vi "AddDependency.vi"(8 "error in (no error)":errorcluster, 9 "Level":string, 10 "Dependency":refnum<class "SMO.lvclass">, 11 "SMO in":refnum<class "SMO.lvclass">) -> (0 "error out":errorcluster, 3 "SMO out":refnum<class "SMO.lvclass">)   [LabVIEW 2013, in "SMO.lvclass"]
uses:
  SMO.lvclass
  Typedefs/SMO Dependency--Cluster.ctl
  Typedefs/SMO Dependency Event--Cluster.ctl
  Typedefs/SMO Dependency Event--Enum.ctl
  SMO.lvclass/SMO.ctl
  <vilib>/regexp/Match Regular Expression.xnode
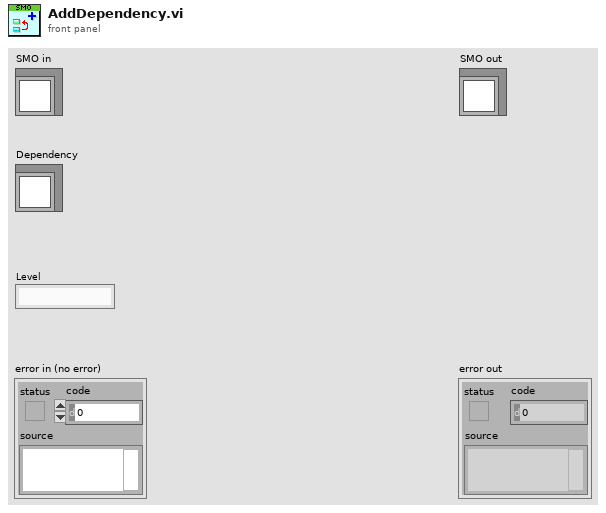
[diagram p1: front panel]
types:
  T1 = typedef "SMO.lvclass/SMO Dependency Event--Cluster.ctl" = cluster{"Name":string, "GUID":string, "Event":T2}
  T2 = typedef "SMO.lvclass/SMO Dependency Event--Enum.ctl" = enum16{"Added", "Removed", "Started", "Stopped"}
  T3 = typedef "SMO.lvclass/SMO Dependency--Cluster.ctl" = cluster{"Dependency":refnum<class "SMO.lvclass">, "Level":string}
  T4 = typedef "SMO.lvclass/PrivateData--Ref.ctl" = refnum<data-value>
  T5 = typedef "SMO.lvclass/PrivateData--Cluster.ctl" = cluster{"Parent Call":T6, "Registered Processes":T7[], "Sync Notifier":refnum<notifier>, "Process Error Notifier":refnum<notifier>, "Protected Events":T8, "Public Events":T9, "SMO State":T10, "[Dependencies]":T3[], "[Attributes]":refnum<class "Attribute.lvclass">[], "Launcher Close":refnum<notifier>, "Caller Watchdog":refnum<queue>}
  T6 = typedef "SMO.lvclass/Parent Call--Enum.ctl" = enum16{"Allows parent to run", "Does not request parent to run"}
  T7 = typedef "SMO.lvclass/RegisteredProcessData--Cluster.ctl" = cluster{"Name":string, "Static VI Ref":refnum<vi>, "Running":bool, "NotifierRef":u32}
  T8 = typedef "SMO.lvclass/Protected Events.ctl" = cluster{"StopProcesses":refnum<user-event>, "AbortProcesses":refnum<user-event>, "Config Changed":refnum<user-event>, "Dependency":refnum<user-event>}
  T9 = typedef "SMO.lvclass/Public Events.ctl" = cluster{"Error":refnum<user-event>, "State":refnum<user-event>}
  T10 = typedef "SMO.lvclass/SMOState --Enum.ctl" = enum16{"unknown", "Created", "Started", "Stopped"}
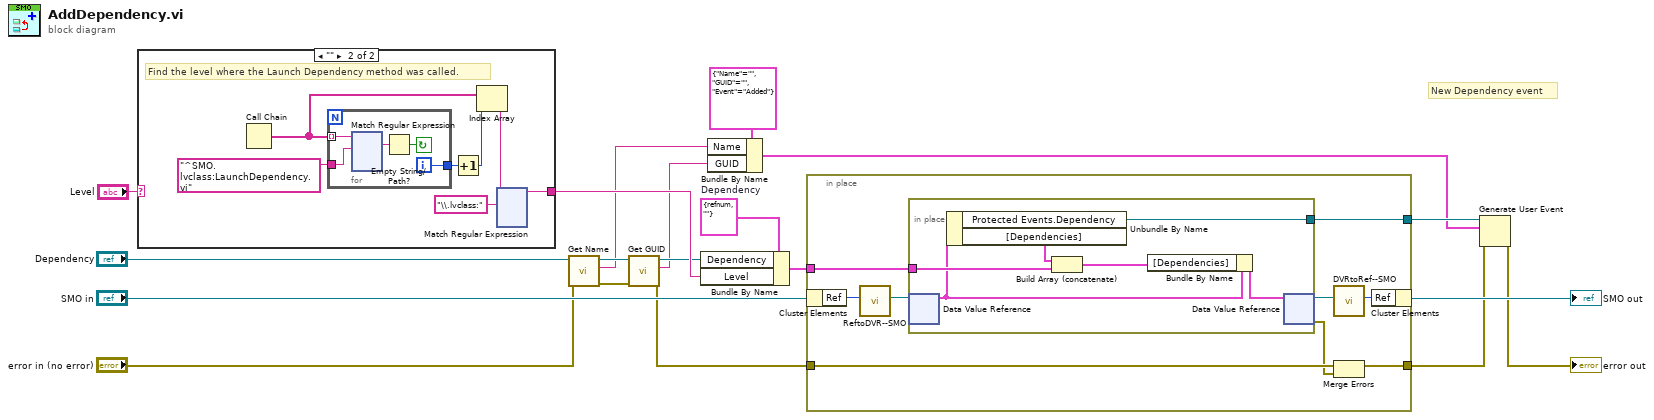
[diagram p0: block diagram]
diagram:
  w18 = T3 {"Dependency"=refnum, "Level"=""}  # Dependency
  # "New Dependency event"
  n1 = case shown="\"\"" "Level" {
    selector: "Level" -> [w20 _]
    tunnel: [w20 w21] -> w16
    frame Default {
    }
    frame "" {
      # "Find the level where the Launch Dependency method was called."
      n2 = Call Chain() -> (call chain=w26:string[])
      n3 = for {
        tunnel: w26 -> [w146] mode=indexing
        tunnel: "^SMO.lvclass:LaunchDependency.vi" -> [w145]
        tunnel: [w142] -> w25
        i -> [w142]
        stop <- w143 continue-if-true
        n4 = xnode "Match Regular Expression"("input string"=w146, "regular expression"=w145) -> ("whole match"=w144:string)  [unwired: 4 in, 4 out]
        n5 = Empty String/Path?(string/path=w144) -> (empty?=w143:bool)
      }
      n6 = Increment(x=w25) -> (x+1=w24:i32)
      n7 = Index Array(array=w26, index=w24) -> (element=w23:string)
      n8 = xnode "Match Regular Expression"("input string"=w23, "regular expression"="\\.lvclass:") -> ("before match"=w21:string)  [unwired: 4 in, 4 out]
    }
  }
  n9 = call "Get Name.vi"("error in (no error)"="error in (no error)", "SMO"="Dependency") -> ("error out"=w8:errorcluster, "Name"=w3:string, "SMO out"=w10:refnum<class "SMO.lvclass">)  [unwired: 7 in]
  n10 = call "Get GUID.vi"("error in (no error)"=w8, "SMO"=w10) -> ("error out"=w5:errorcluster, "GUID"=w2:string, "SMO out"=w9:refnum<class "SMO.lvclass">)  [unwired: 7 in]
  n11 = Bundle By Name(cluster=w18, "Dependency"=w9, "Level"=w16) -> (w17:T3)
  n12 = Bundle By Name(cluster=T1 {"Name"="", "GUID"="", "Event"=enum."Added"} ("Dependency Event"), "Name"=w3, "GUID"=w2) -> (w1:T1)
  n13 = in-place {
    in-place-border: w5 -> [w265]
    in-place-border: [w263] -> w12
    in-place-border: w17 -> [w262]
    in-place-border: [w261] -> w14
    n14 = in-place-cluster #1("SMO in") -> ("Ref"=w269:u32)
    n15 = call "ReftoDVR--SMO.vi"("Ref"=w269) -> ("Ref"=w268:T4)  [unwired: 10 in]
    n16 = in-place {
      in-place-border: w262 -> [w273]
      in-place-border: [w270] -> w261
      n17 = in-place-dvr #2(w268) -> (w271:T5)  [unwired: 1 out]
      n18 = Unbundle By Name(w271) -> ("Protected Events.Dependency"=w270:refnum<user-event>, "[Dependencies]"=w274:T3[])
      n19 = Build Array (concatenate)(w274, w273) -> (w272:T3[])
      n20 = Bundle By Name(cluster=w271, "[Dependencies]"=w272) -> (w275:T5)
      n21 = in-place-dvr #2(w275) -> (w267:T4, w264:errorcluster)
    }
    n22 = call "DVRtoRef--SMO.vi"("Ref"=w267) -> ("Ref"=w266:u32)  [unwired: 10 in]
    n23 = Merge Errors(w265, w264) -> (w263:errorcluster)
    n24 = in-place-cluster #1("Ref"=w266) -> (→"SMO out":refnum<class "SMO.lvclass">)
  }
  n25 = Generate User Event(user event=w14, event data cluster=w1, error in=w12) -> (error out=→"error out":errorcluster)  [unwired: 1 in, 1 out]
